vi "interfaz1.vi"() -> ()   [LabVIEW 2020]
panel:
  out "read buffer":string
  in  "VISA resource name":refnum<visa-resource-name>
  in  "stop":bool
  out "Thermometer":dbl(slide) scale=0.0..100.0
  out "Waveform Chart":dbl[][](graph)
  # "Instituto Politécnico Nacional \nEscuela Superior de Cómputo\nInstrumentación \nSistema de Medición Virtual"
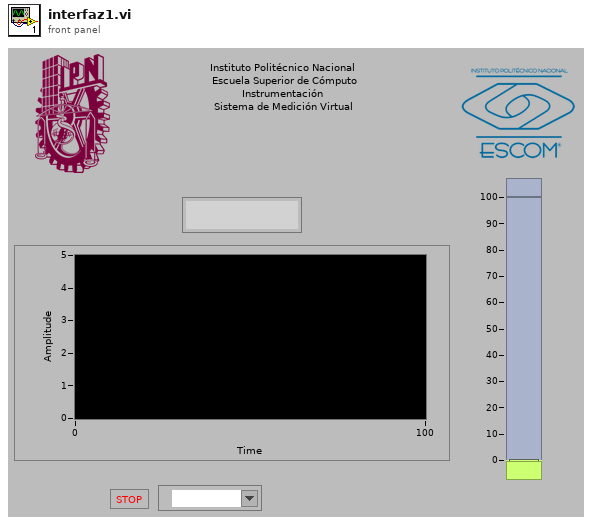
[diagram p1: front panel]
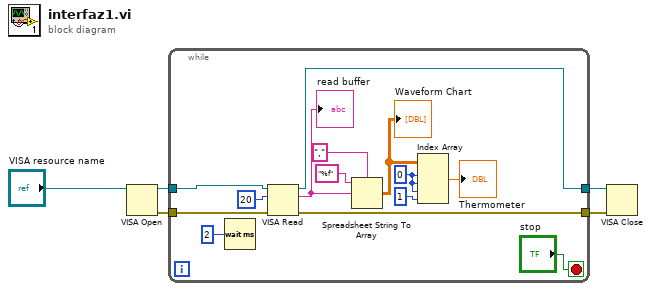
[diagram p0: block diagram]
diagram:
  n1 = VISA Open(VISA resource name="VISA resource name") -> (VISA resource name=w5:refnum<visa-resource-name>, error out=w4:errorcluster)  [unwired: 4 in]
  n2 = while {
    tunnel: w5 -> [w19]
    tunnel: w4 -> [w18]
    tunnel: [w17] -> w3
    tunnel: [w15] -> w2
    stop <- "stop" stop-if-true
    w6 = 0 ("index (row)")
    n3 = Wait (ms)(milliseconds to wait=u32 2) -> ()  [unwired: 1 out]
    n4 = VISA Read(VISA resource name=w19, byte count=u32 20, error in (no error)=w18) -> (VISA resource name out=w17:refnum<visa-resource-name>, read buffer=w9:string, error out=w15:errorcluster)  [unwired: 1 out]
    "read buffer" <- w9
    n5 = Spreadsheet String To Array(delimiter (Tab)=",", format string="%f", spreadsheet string=w9) -> (array=w8:dbl[][])  [unwired: 1 in]
    "Waveform Chart" <- w8
    n6 = Index Array(array=w8, index (row) #1=w6, index (col) #1=w6, index (row) #2=w6, index (col) #2=1 ("index (col)")) -> (element #1=→"Thermometer":dbl)  [unwired: 1 out]
  }
  n7 = VISA Close(VISA resource name=w3, error in (no error)=w2) -> ()  [unwired: 1 out]
